vi "QualityOfLifeShit.vi"() -> ()   [LabVIEW 2021]
uses:
  <userlib>/Nanonis Prog Interface V5/Nanonis Prog Interface.lvlib
panel:
  in  "?":T1(tab)
  in  "Scan Frame \nSize (m)":dbl=2e-09 format="%#_6p"
  in  "Scan Frame":bool
  in  "Lockin frequency":dbl=1000.0
  out "Capacitance after (pA)":dbl
  out "Capacitance before (pA)":dbl
  out "Didn't walk out?":bool
  out "Delta capacitance (pA)":dbl
  in  "Walk out":bool
  in  "Walk out Amplitude (V)":sgl=370.0
  in  "Walk out steps per set":u16=10
  in  "Number of sets of steps":i32=7
  in  "Coordinates\nAmplitude (V)":dbl=1.0
  in  "Coordinates \nFrequency (Hz)":dbl=1000.0
  in  "Navigation \nAmplitude (V)":dbl=1.5
  in  "Navigation \nFrequency (Hz)":dbl=3886.7
  in  "Turn on":bool
  in  "Turn off":bool
  in  "Coordinates":bool
  in  "Navigation":bool
  in  "Stop approach":bool
  in  "Approach voltage":dbl=220.0
  in  "Approach":bool
  in  "Amplitude (V)":dbl=0.01
  in  "Frequency (Hz)":dbl=381.7
  in  "Set lockin \nparameters":bool
  in  "Zero Bias":bool
  # "to Tip"
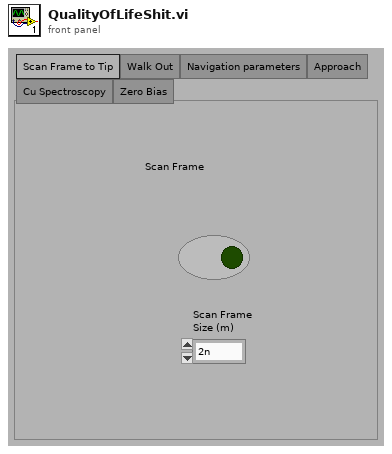
[diagram p1: front panel]
types:
  T1 = enum32{"Scan Frame to Tip", "Walk Out", "Navigation parameters", "Approach", "Cu Spectroscopy", "Zero Bias"}
  T2 = cluster{"Scan Frame \nSize (m)":dbl, "Scan Frame \nSize (m)":dbl}
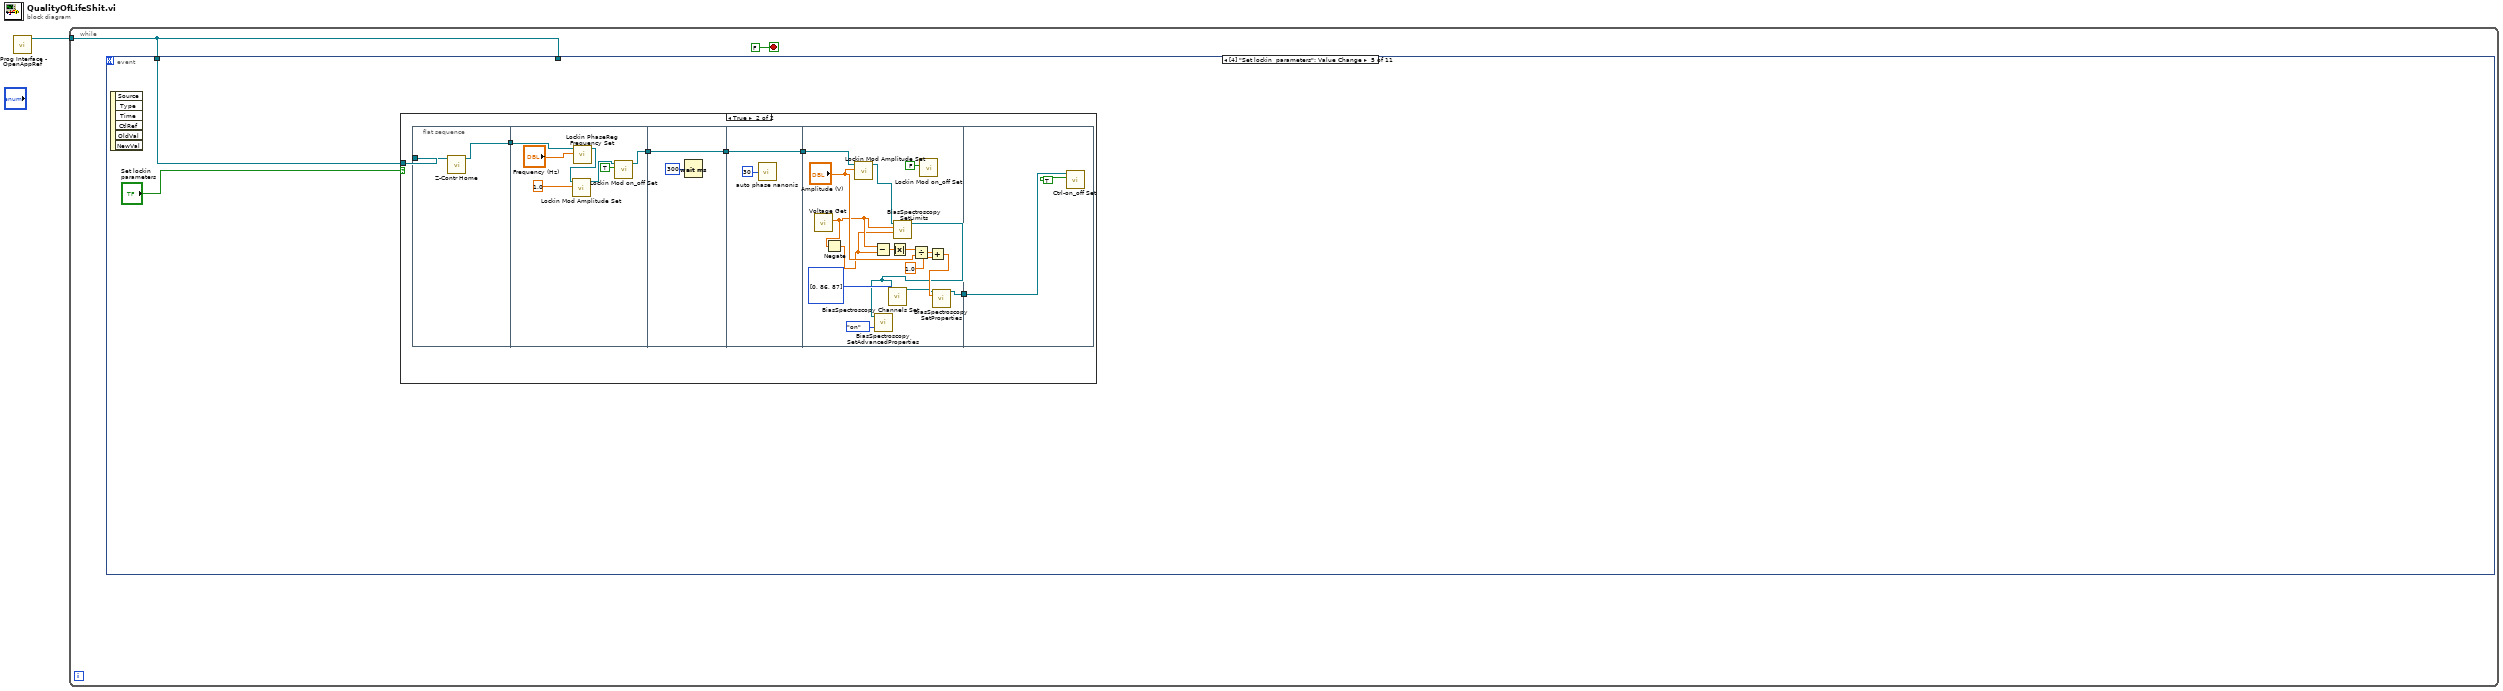
[diagram p0: block diagram]
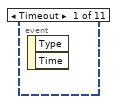
[diagram p2: hidden frame]
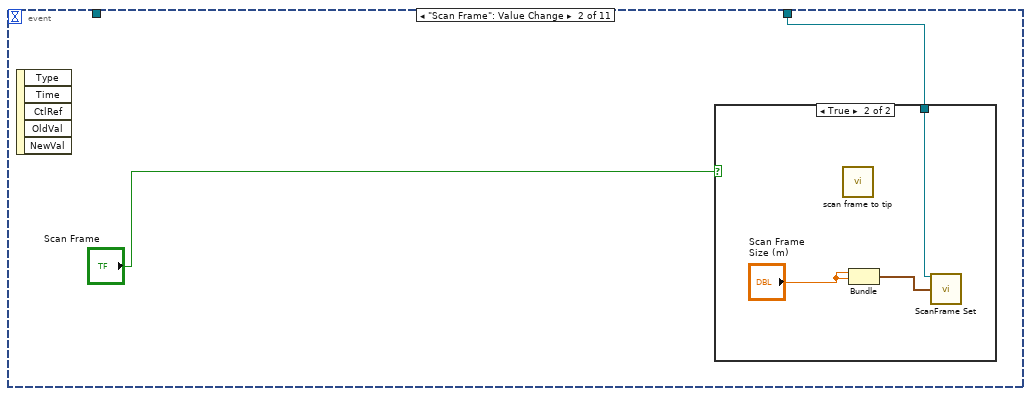
[diagram p3: hidden frame]
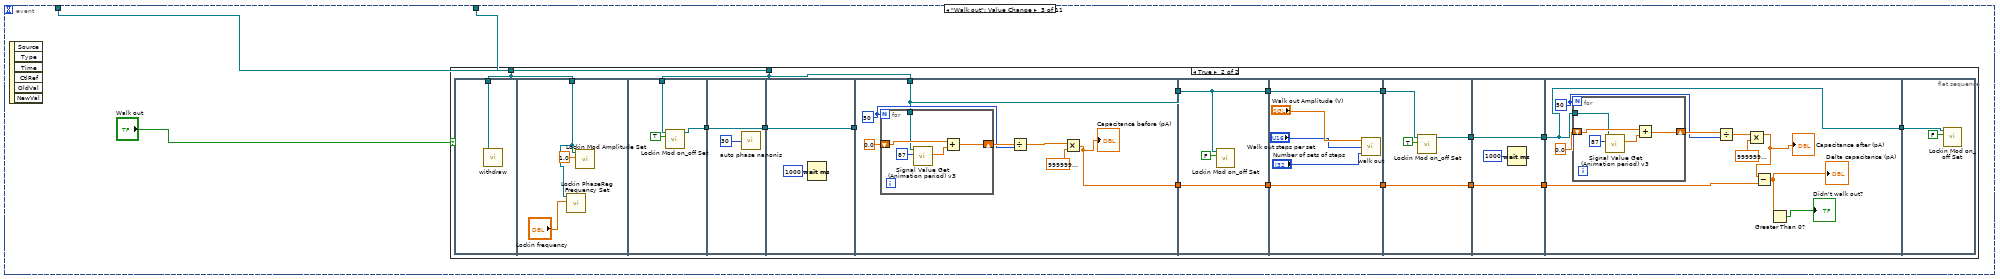
[diagram p5: hidden frame]
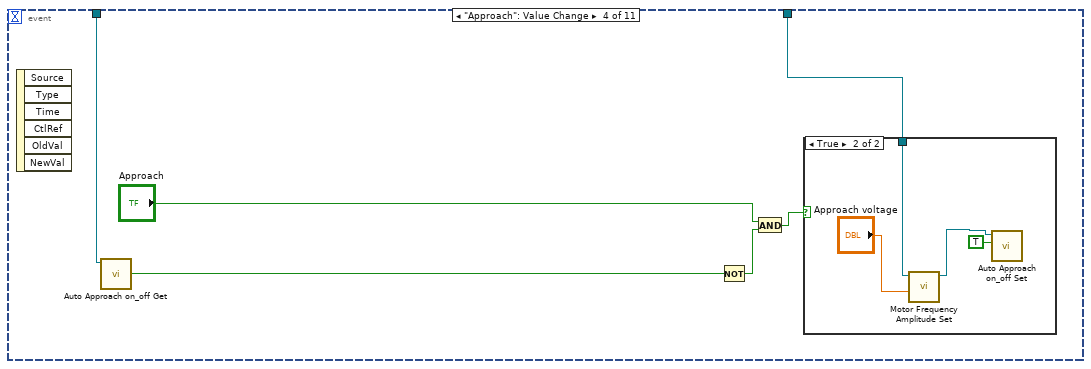
[diagram p7: hidden frame]
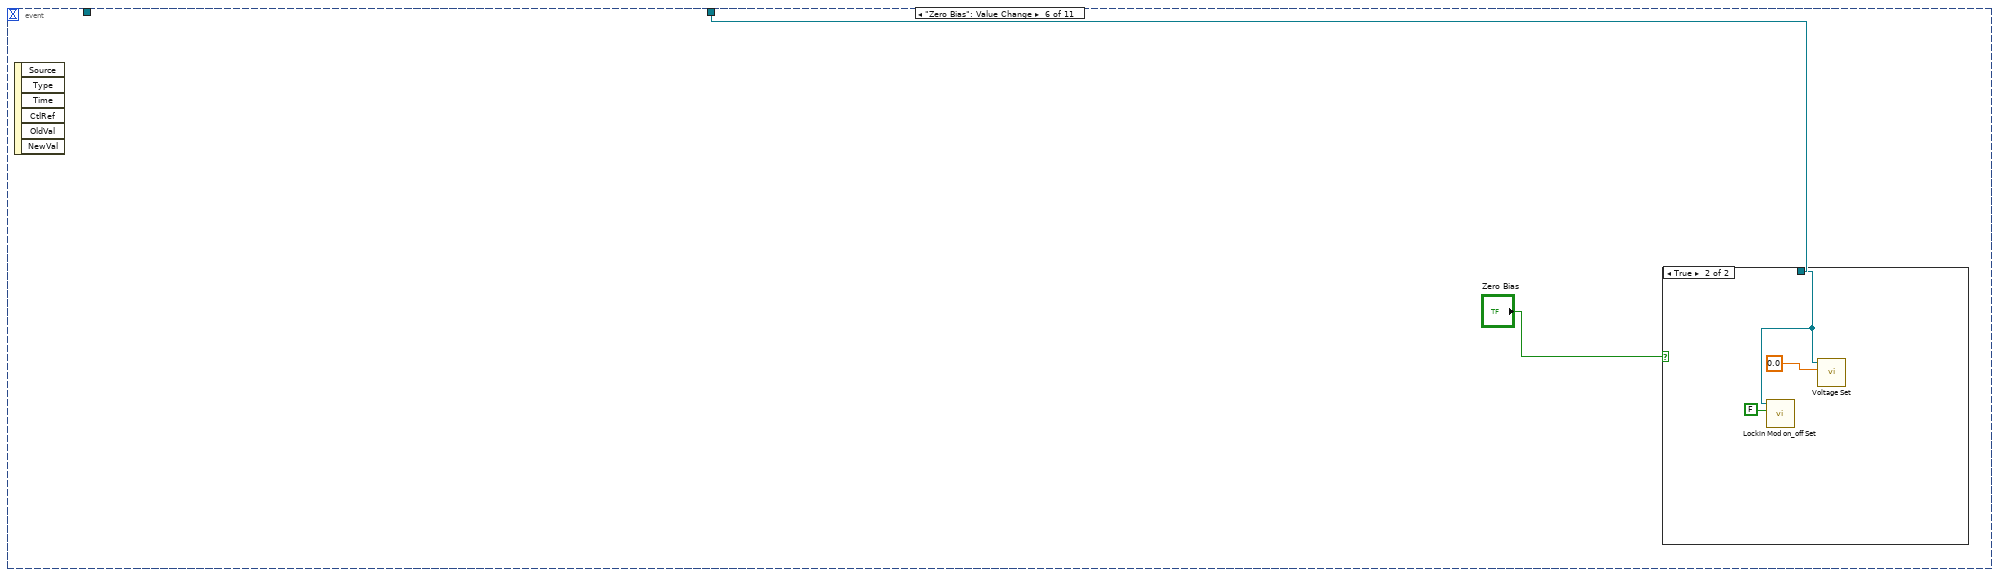
[diagram p10: hidden frame]
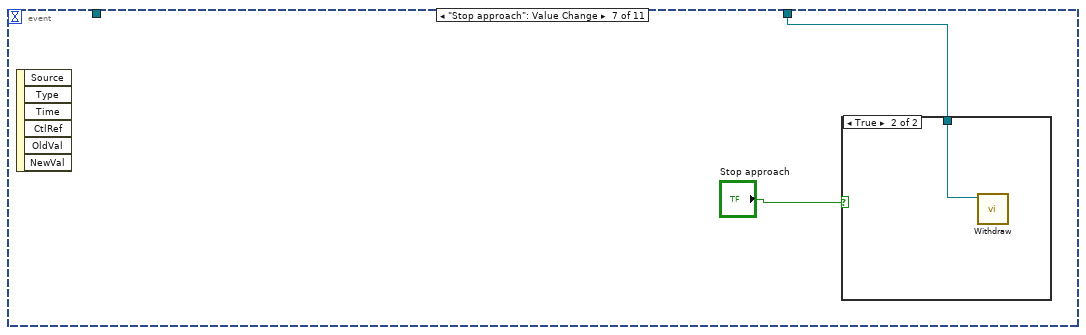
[diagram p12: hidden frame]
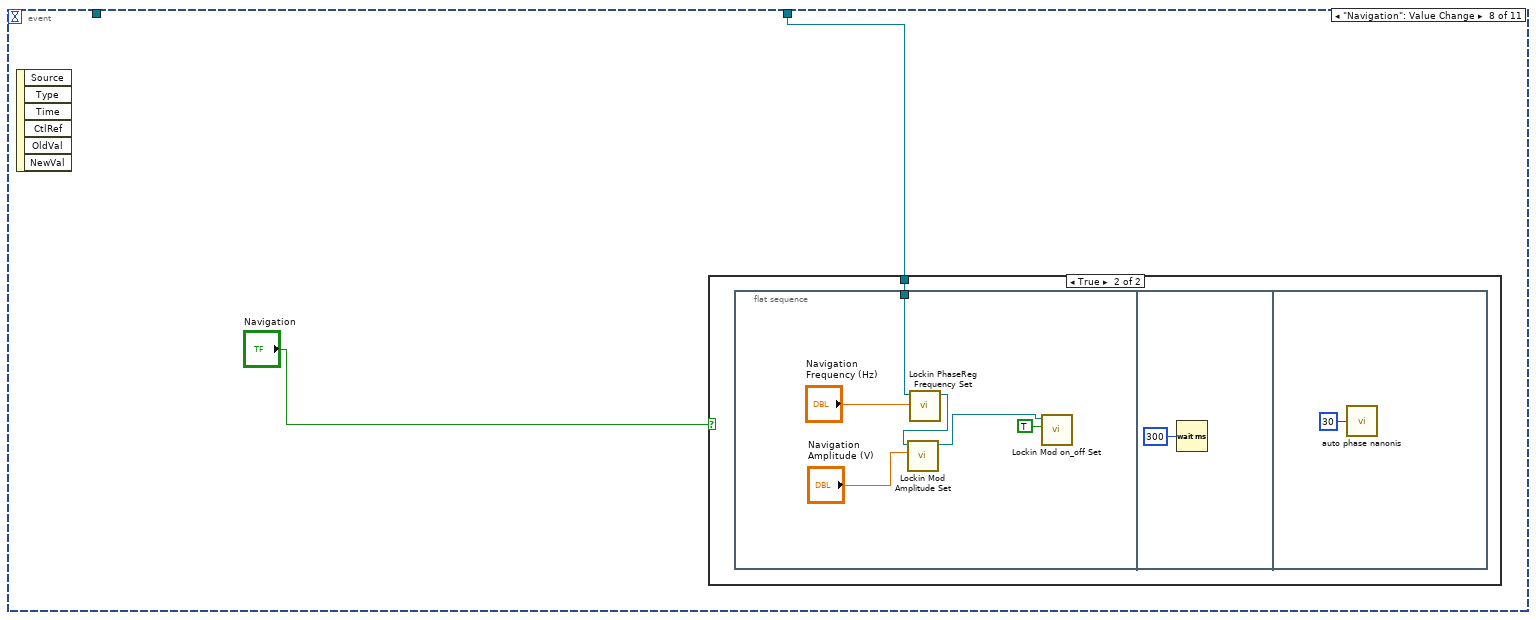
[diagram p14: hidden frame]
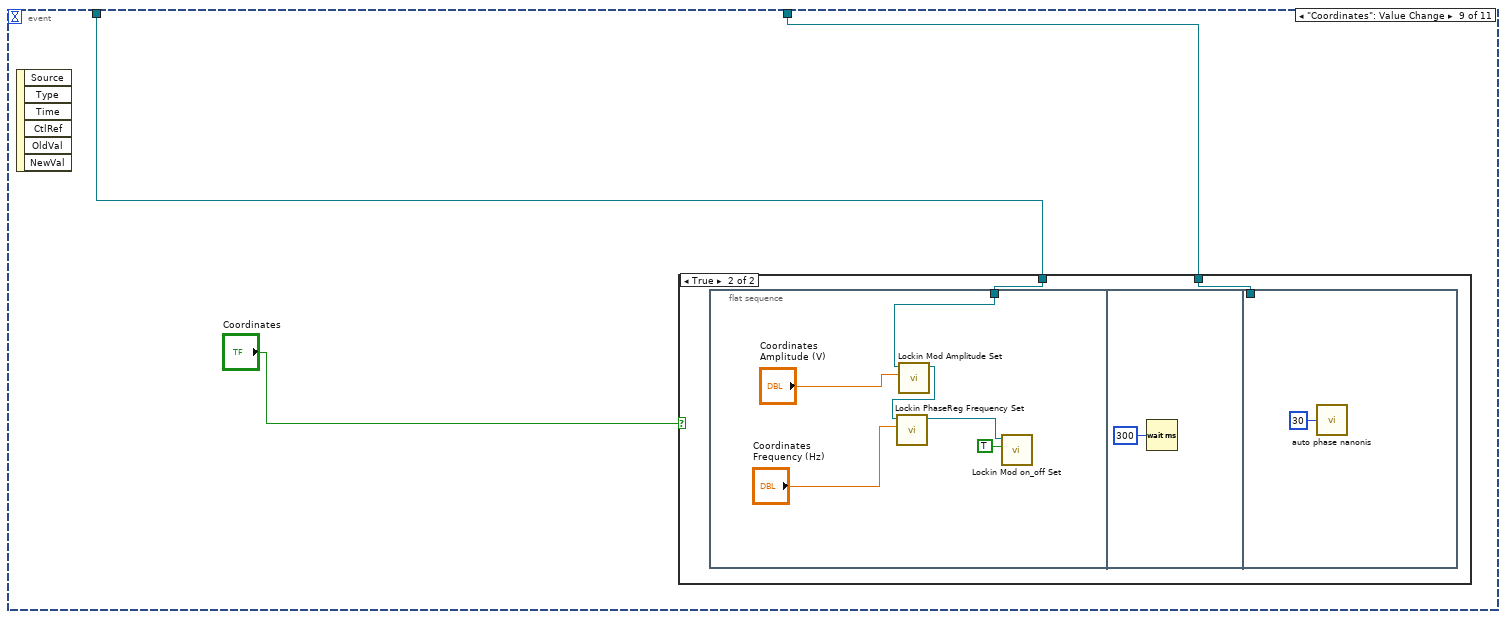
[diagram p16: hidden frame]
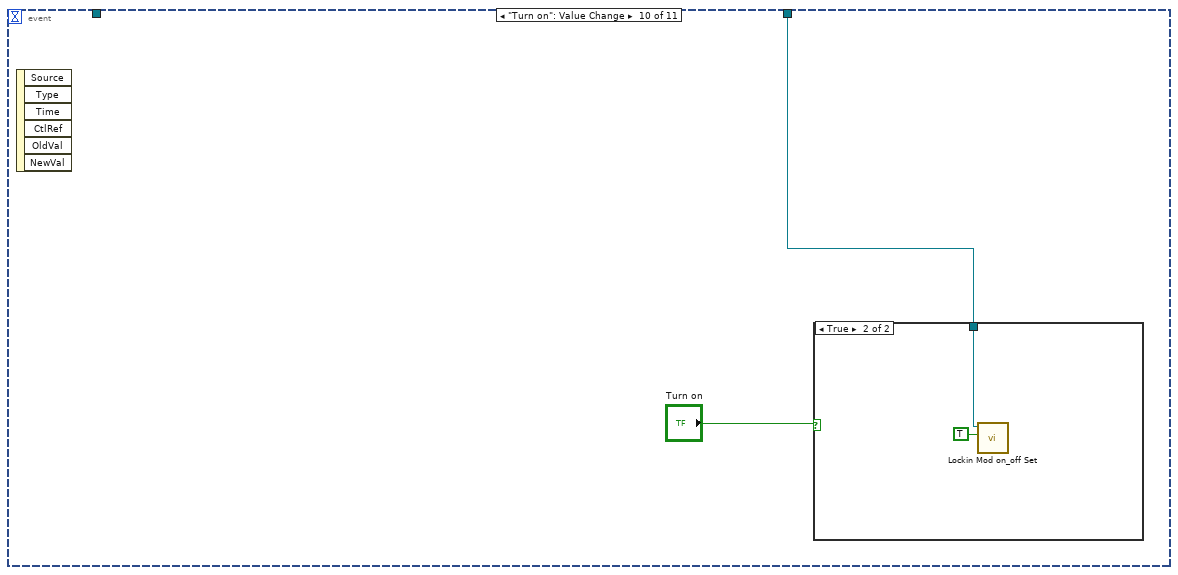
[diagram p18: hidden frame]
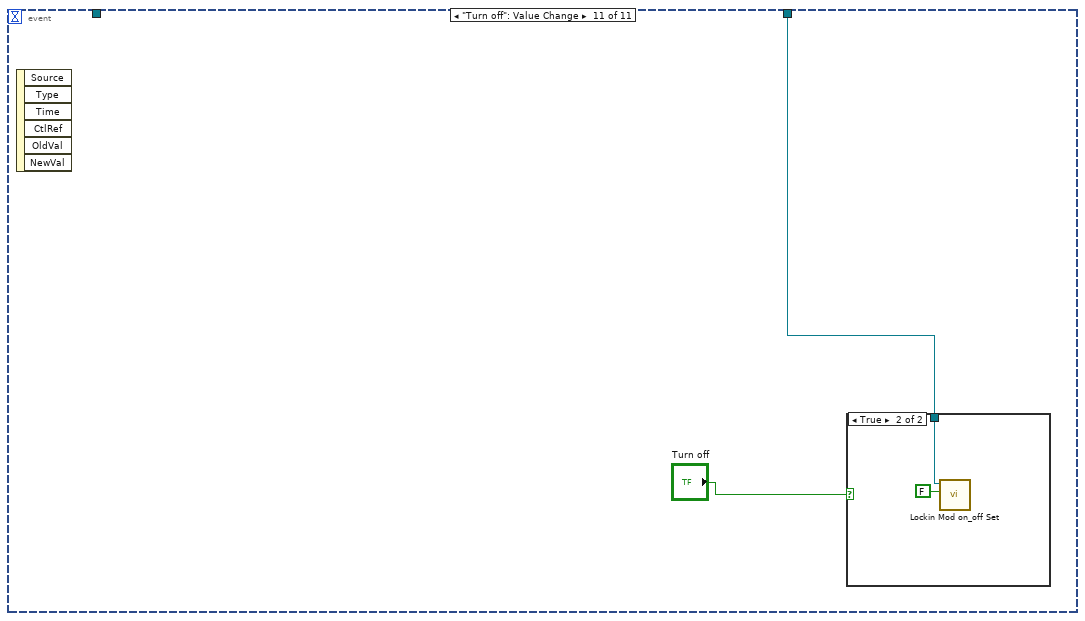
[diagram p20: hidden frame]
diagram:
  n1 = call <userlib>:"Prog Interface - OpenAppRef.vi"() -> ("Application reference"=w1:refnum<vi>)  [unwired: 6 in, 1 out]
  n2 = while {
    tunnel: w1 -> [w2]
    stop <- FALSE stop-if-true
    n3 = event shown="[4] \"Set lockin  parameters\": Value Change" {
      selector: _ -> [_ _ _ _ _ _ _ _ _ _ _]
      dyn-events: _ -> [_ _ _ _ _ _ _ _ _ _ _]
      timeout: _ -> [_ _ _ _ _ _ _ _ _ _ _]
      tunnel: w2 -> [_ w4 w10 w88 _ w132 w137 w140 w152 w164 w168]
      tunnel: w2 -> [_ _ w9 w83 w93 _ _ _ w153 _ _]
      event Timeout {
        n4 = event-data() -> ()  [unwired: 1 in, 2 out]
      }
      event "Scan Frame": Value Change {
        n5 = event-data() -> ()  [unwired: 1 in, 5 out]
        n6 = case shown="True" "Scan Frame" {
          tunnel: w4 -> [_ w6]
          frame False {
          }
          frame True {
            n7 = call "scan frame to tip.vi"() -> ()  [unwired: 12 in]
            n8 = Bundle("Scan Frame \nSize (m)"="Scan Frame \nSize (m)", "Scan Frame \nSize (m)"="Scan Frame \nSize (m)") -> (w7:T2)  [unwired: 1 in]
            n9 = call <userlib>:"ScanFrame Set.vi"("Application ref in"=w6, "Size (m)"=w7) -> ()  [unwired: 12 in, 2 out]
          }
        }
      }
      event "Walk out": Value Change {
        n10 = event-data() -> ()  [unwired: 1 in, 6 out]
        n11 = case shown="True" "Walk out" {
          tunnel: w10 -> [_ w27]
          tunnel: w9 -> [_ w12]
          frame False {
          }
          frame True {
            n12 = flat-sequence {
              tunnel: w12 -> [w28]
              tunnel: w12 -> [w30]
              tunnel: w27 -> [w33]
              tunnel: [w32] -> w26
              tunnel: [w35] -> w18
              tunnel: w26 -> [w35]
              tunnel: w18 -> [w38]
              tunnel: [w38] -> w17
              tunnel: [w39] -> w22
              tunnel: w27 -> [w43]
              tunnel: [w43] -> w20
              tunnel: w17 -> [_]
              tunnel: w22 -> [w53]
              tunnel: [w53] -> w21
              tunnel: w20 -> [w51]
              tunnel: [w51] -> w19
              tunnel: [w55] -> w25
              tunnel: w21 -> [w55]
              tunnel: [w54] -> w24
              tunnel: w19 -> [w54]
              tunnel: w25 -> [w62]
              tunnel: [w62] -> w16
              tunnel: w24 -> [w60]
              tunnel: [w59] -> w14
              tunnel: w16 -> [w65]
              tunnel: [w65] -> w15
              tunnel: w14 -> [w64]
              tunnel: [w64] -> w13
              tunnel: w15 -> [w72]
              tunnel: w13 -> [w71]
              tunnel: [w71] -> w23
              tunnel: w23 -> [w81]
              frame #0 {
                n13 = call <userlib>:"withdraw.vi"("Application ref in"=w28) -> ()  [unwired: 2 in, 1 out]
              }
              frame #1 {
                n14 = call <userlib>:"Lockin PhaseReg Frequency Set.vi"("Frequency (Hz)"="Lockin frequency", "Application ref in"=w30) -> ()  [unwired: 8 in, 2 out]
                n15 = call <userlib>:"Lockin Mod Amplitude Set.vi"("Amplitude (mod. signal unit)"=sgl 1.0, "Application ref in"=w30) -> ()  [unwired: 8 in, 2 out]
              }
              frame #2 {
                n16 = call <userlib>:"Lockin Mod on_off Set.vi"("Lockin ON/OFF"=TRUE, "Application ref in"=w33) -> ("Application ref out"=w32:refnum<vi>)  [unwired: 8 in, 1 out]
              }
              frame #3 {
                n17 = call "auto phase nanonis.vi"("Num averages"=u32 30) -> ()
              }
              frame #4 {
                n18 = Wait (ms)(milliseconds to wait=u32 1000) -> ()  [unwired: 1 out]
              }
              frame #5 {
                w44 = 50
                n19 = for {
                  N: w44 -> [_]
                  shift-right: [w48] -> w45
                  shift-left: sgl 0.0 -> [w47]
                  tunnel: w43 -> [w46]
                  n20 = call <userlib>:"Signal Value Get (Animation period) v3.vi"("Signal index (0-127)"=i8 87, "Application ref in"=w46) -> ("Signal value"=w49:sgl)  [unwired: 6 in, 2 out]
                  n21 = Add(x=w47, y=w49) -> (x+y=w48:sgl)
                }
                n22 = Divide(x=w45, y=w44) -> (x/y=w42:sgl)
                n23 = Multiply(x=w42, y=sgl 1000000000000.0) -> (x*y=w39:sgl)
                "Capacitance before (pA)" <- w39
              }
              frame #6 {
                n24 = call <userlib>:"Lockin Mod on_off Set.vi"("Lockin ON/OFF"=FALSE, "Application ref in"=w51) -> ()  [unwired: 8 in, 2 out]
              }
              frame #7 {
                n25 = call "walk out.vi"("Number of sets of steps"="Number of sets of steps", "Walk out number steps"="Walk out steps per set", "Walk out Amplitude (V)"="Walk out Amplitude (V)") -> ()
              }
              frame #8 {
                n26 = call <userlib>:"Lockin Mod on_off Set.vi"("Lockin ON/OFF"=TRUE, "Application ref in"=w60) -> ("Application ref out"=w59:refnum<vi>)  [unwired: 8 in, 1 out]
              }
              frame #9 {
                n27 = Wait (ms)(milliseconds to wait=u32 1000) -> ()  [unwired: 1 out]
              }
              frame #10 {
                w74 = 50
                n28 = for {
                  N: w74 -> [_]
                  shift-right: [w78] -> w75
                  shift-left: sgl 0.0 -> [w77]
                  tunnel: w71 -> [w76]
                  n29 = call <userlib>:"Signal Value Get (Animation period) v3.vi"("Signal index (0-127)"=i8 87, "Application ref in"=w76) -> ("Signal value"=w79:sgl)  [unwired: 6 in, 2 out]
                  n30 = Add(x=w77, y=w79) -> (x+y=w78:sgl)
                }
                n31 = Divide(x=w75, y=w74) -> (x/y=w73:sgl)
                n32 = Multiply(x=w73, y=sgl 1000000000000.0) -> (x*y=w66:sgl)
                "Capacitance after (pA)" <- w66
                n33 = Subtract(x=w66, y=w72) -> (x-y=w70:sgl)
                "Delta capacitance (pA)" <- w70
                n34 = Greater Than 0?(x=w70) -> (x > 0?=→"Didn't walk out?":bool)
              }
              frame #11 {
                n35 = call <userlib>:"Lockin Mod on_off Set.vi"("Lockin ON/OFF"=FALSE, "Application ref in"=w81) -> ()  [unwired: 8 in, 2 out]
              }
            }
          }
        }
      }
      event "Approach": Value Change {
        n36 = event-data() -> ()  [unwired: 1 in, 6 out]
        n37 = call <userlib>:"Auto Approach on_off Get.vi"("Application ref in"=w83) -> ("Auto approach on/off status"=w87:bool)  [unwired: 6 in, 2 out]
        n38 = Not(x=w87) -> (.not. x?=w85:bool)
        n39 = And(x="Approach", y=w85) -> (x .and. y?=w86:bool)
        n40 = case shown="True" w86 {
          tunnel: w88 -> [_ w90]
          frame False {
          }
          frame True {
            n41 = call <userlib>:"Motor Frequency Amplitude Set.vi"("Amplitude (V) (NaN=no change)"="Approach voltage", "Application ref in"=w90) -> ("Application ref out"=w89:refnum<vi>)  [unwired: 8 in, 1 out]
            n42 = call <userlib>:"Auto Approach on_off Set.vi"("Auto approach start/stop (F)"=TRUE, "Application ref in"=w89) -> ()  [unwired: 6 in, 2 out]
          }
        }
      }
      event "Set lockin \nparameters": Value Change {
        n43 = event-data() -> ()  [unwired: 1 in, 6 out]
        n44 = case shown="True" "Set lockin \nparameters" {
          tunnel: w93 -> [_ w100]
          frame False {
          }
          frame True {
            n45 = flat-sequence {
              tunnel: w100 -> [w102]
              tunnel: [w101] -> w99
              tunnel: w99 -> [w106]
              tunnel: [w103] -> w97
              tunnel: [w110] -> w98
              tunnel: w97 -> [w110]
              tunnel: [w112] -> w96
              tunnel: w98 -> [w112]
              tunnel: w96 -> [w129]
              tunnel: [w121] -> w95
              tunnel: w95 -> [w130]
              frame #0 {
                n46 = call <userlib>:"Z-Contr Home.vi"("Application ref in"=w102) -> ("Application ref out"=w101:refnum<vi>)  [unwired: 9 in, 1 out]
              }
              frame #1 {
                n47 = call <userlib>:"Lockin PhaseReg Frequency Set.vi"("Frequency (Hz)"="Frequency (Hz)", "Application ref in"=w106) -> ("Application ref out"=w105:refnum<vi>)  [unwired: 8 in, 1 out]
                n48 = call <userlib>:"Lockin Mod Amplitude Set.vi"("Amplitude (mod. signal unit)"=sgl 1.0, "Application ref in"=w105) -> ("Application ref out"=w104:refnum<vi>)  [unwired: 8 in, 1 out]
                n49 = call <userlib>:"Lockin Mod on_off Set.vi"("Lockin ON/OFF"=TRUE, "Application ref in"=w104) -> ("Application ref out"=w103:refnum<vi>)  [unwired: 8 in, 1 out]
              }
              frame #2 {
                n50 = Wait (ms)(milliseconds to wait=u32 300) -> ()  [unwired: 1 out]
              }
              frame #3 {
                n51 = call "auto phase nanonis.vi"("Num averages"=u32 30) -> ()
              }
              frame #4 {
                n52 = call <userlib>:"Voltage Get.vi"() -> ("Bias (V)"=w120:sgl)  [unwired: 9 in, 2 out]
                n53 = Negate(x=w120) -> (-x=w119:sgl)
                n54 = call <userlib>:"Lockin Mod Amplitude Set.vi"("Amplitude (mod. signal unit)"="Amplitude (V)", "Application ref in"=w129) -> ("Application ref out"=w128:refnum<vi>)  [unwired: 8 in, 1 out]
                n55 = Subtract(x=w120, y=w119) -> (x-y=w127:sgl)
                n56 = Absolute Value(x=w127) -> (abs(x)=w126:sgl)
                n57 = call <userlib>:"BiasSpectroscopy SetLimits.vi"("End value (V)"=w119, "Start value (V)"=w120, "Application ref in"=w128) -> ("Application ref out"=w116:refnum<vi>)  [unwired: 5 in, 1 out]
                n58 = call <userlib>:"BiasSpectroscopy SetAdvancedProperties.vi"("Application ref in"=w116, "Lockin run (no change)"=enum16{"no change", "on", "off"}."on") -> ()  [unwired: 12 in, 2 out]
                n59 = call <userlib>:"BiasSpectroscopy Channels Set.vi"("Channels"=i8[] [0, 86, 87], "Application ref in"=w116) -> ("Application ref out"=w117:refnum<vi>)  [unwired: 8 in, 1 out]
                n60 = Divide(x=w126, y="Amplitude (V)") -> (x/y=w124:dbl)
                n61 = call <userlib>:"Lockin Mod on_off Set.vi"("Lockin ON/OFF"=FALSE) -> ()  [unwired: 9 in, 2 out]
                n62 = Add(x=w124, y=1.0) -> (x+y=w122:dbl)
                n63 = call <userlib>:"BiasSpectroscopy SetProperties.vi"("Application ref in"=w117, "Number of points (0=no change)"=w122) -> ("Application ref out"=w121:refnum<vi>)  [unwired: 12 in, 1 out]
              }
              frame #5 {
                n64 = call <userlib>:"Ctrl-on_off Set.vi"("Z Controller ON/OFF"=TRUE, "Application ref in"=w130) -> ()  [unwired: 8 in, 2 out]
              }
            }
          }
        }
      }
      event "Zero Bias": Value Change {
        n65 = event-data() -> ()  [unwired: 1 in, 6 out]
        n66 = case shown="True" "Zero Bias" {
          tunnel: w132 -> [_ w134]
          frame False {
          }
          frame True {
            n67 = call <userlib>:"Lockin Mod on_off Set.vi"("Lockin ON/OFF"=FALSE, "Application ref in"=w134) -> ()  [unwired: 8 in, 2 out]
            n68 = call <userlib>:"Voltage Set.vi"("Bias (V)"=sgl 0.0, "Application ref in"=w134) -> ()  [unwired: 8 in, 2 out]
          }
        }
      }
      event "Stop approach": Value Change {
        n69 = event-data() -> ()  [unwired: 1 in, 6 out]
        n70 = case shown="True" "Stop approach" {
          tunnel: w137 -> [_ w139]
          frame False {
          }
          frame True {
            n71 = call <userlib>:"Withdraw.vi"("Application ref in"=w139) -> ()  [unwired: 9 in, 2 out]
          }
        }
      }
      event "Navigation": Value Change {
        n72 = event-data() -> ()  [unwired: 1 in, 6 out]
        n73 = case shown="True" "Navigation" {
          tunnel: w140 -> [_ w142]
          frame False {
          }
          frame True {
            n74 = flat-sequence {
              tunnel: w142 -> [w145]
              frame #0 {
                n75 = call <userlib>:"Lockin PhaseReg Frequency Set.vi"("Frequency (Hz)"="Navigation \nFrequency (Hz)", "Application ref in"=w145) -> ("Application ref out"=w148:refnum<vi>)  [unwired: 8 in, 1 out]
                n76 = call <userlib>:"Lockin Mod Amplitude Set.vi"("Amplitude (mod. signal unit)"="Navigation \nAmplitude (V)", "Application ref in"=w148) -> ("Application ref out"=w146:refnum<vi>)  [unwired: 8 in, 1 out]
                n77 = call <userlib>:"Lockin Mod on_off Set.vi"("Lockin ON/OFF"=TRUE, "Application ref in"=w146) -> ()  [unwired: 8 in, 2 out]
              }
              frame #1 {
                n78 = Wait (ms)(milliseconds to wait=u32 300) -> ()  [unwired: 1 out]
              }
              frame #2 {
                n79 = call "auto phase nanonis.vi"("Num averages"=u32 30) -> ()
              }
            }
          }
        }
      }
      event "Coordinates": Value Change {
        n80 = event-data() -> ()  [unwired: 1 in, 6 out]
        n81 = case shown="True" "Coordinates" {
          tunnel: w153 -> [_ w155]
          tunnel: w152 -> [_ w154]
          frame False {
          }
          frame True {
            n82 = flat-sequence {
              tunnel: w155 -> [w161]
              tunnel: w154 -> [_]
              frame #0 {
                n83 = call <userlib>:"Lockin Mod Amplitude Set.vi"("Amplitude (mod. signal unit)"="Coordinates\nAmplitude (V)", "Application ref in"=w161) -> ("Application ref out"=w160:refnum<vi>)  [unwired: 8 in, 1 out]
                n84 = call <userlib>:"Lockin PhaseReg Frequency Set.vi"("Frequency (Hz)"="Coordinates \nFrequency (Hz)", "Application ref in"=w160) -> ("Application ref out"=w158:refnum<vi>)  [unwired: 8 in, 1 out]
                n85 = call <userlib>:"Lockin Mod on_off Set.vi"("Lockin ON/OFF"=TRUE, "Application ref in"=w158) -> ()  [unwired: 8 in, 2 out]
              }
              frame #1 {
                n86 = Wait (ms)(milliseconds to wait=u32 300) -> ()  [unwired: 1 out]
              }
              frame #2 {
                n87 = call "auto phase nanonis.vi"("Num averages"=u32 30) -> ()
              }
            }
          }
        }
      }
      event "Turn on": Value Change {
        n88 = event-data() -> ()  [unwired: 1 in, 6 out]
        n89 = case shown="True" "Turn on" {
          tunnel: w164 -> [_ w167]
          frame False {
          }
          frame True {
            n90 = call <userlib>:"Lockin Mod on_off Set.vi"("Lockin ON/OFF"=TRUE, "Application ref in"=w167) -> ()  [unwired: 8 in, 2 out]
          }
        }
      }
      event "Turn off": Value Change {
        n91 = event-data() -> ()  [unwired: 1 in, 6 out]
        n92 = case shown="True" "Turn off" {
          tunnel: w168 -> [_ w170]
          frame False {
          }
          frame True {
            n93 = call <userlib>:"Lockin Mod on_off Set.vi"("Lockin ON/OFF"=FALSE, "Application ref in"=w170) -> ()  [unwired: 8 in, 2 out]
          }
        }
      }
    }
  }
